vi "E_pressure_read_multiple_channels.vi"(3 "error in":errorcluster, 4 "Test Array":dbl[](array[numeric]), 5 "Test Mode":bool) -> (0 "error out":errorcluster, 1 "Scaled Pressures":dbl[](array[numeric]))   [LabVIEW 2013]
uses:
  <vilib>/DAQmx/read.llb/DAQmx Read (Analog 1D Wfm NChan NSamp).vi
  <vilib>/Analysis/baseanly.llb/Mean (DBL).vi
  <vilib>/DAQmx/miscellaneous.llb/DAQmx Fill In Error Info.vi
  <vilib>/Analysis/NI_AALBase.lvlib
panel:
  out "Raw Input Voltage":dbl[](array[numeric])
  out "data":waveform(dbl)[](graph)
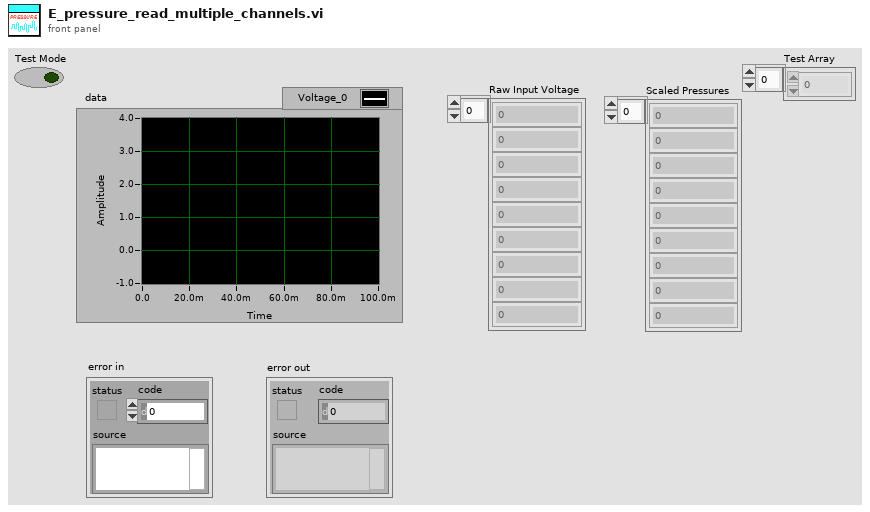
[diagram p1: front panel]
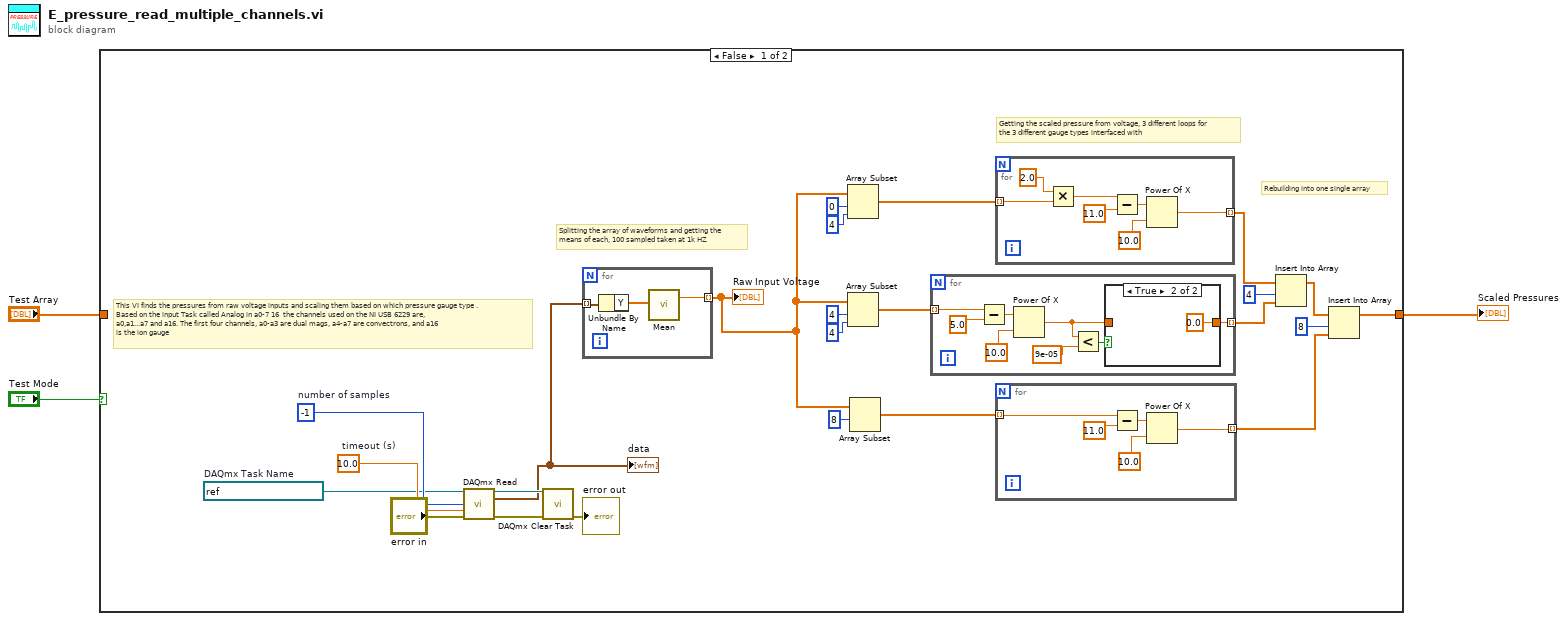
[diagram p0: block diagram]
diagram:
  n1 = case shown="False" "Test Mode" {
    tunnel: [w7 w53] -> w3
    tunnel: "Test Array" -> [_ w53]
    frame False {
      w23 = refnum<k21> "Analog in a0-7 16"  # DAQmx Task Name
      w26 = 10.0  # timeout (s)
      w27 = -1  # number of samples
      # "Rebuilding into one single array"
      # "Splitting the array of waveforms and getting the\nmeans of each, 100 sampled taken at 1k HZ"
      # "Getting the scaled pressure from voltage, 3 different loops for\nthe 3 different gauge types interfaced with"
      # "This VI finds the pressures from raw voltage inputs and scaling them based on which pressure gauge type .\nBased on the input Task called Analog in a0-7 16  the channels used on the NI USB 6229 are,\na0,a1...a7 and a16. The first four channels, a0-a3 are dual mags, a4-a7 are convectrons, and a16\nis the ion gauge"
      n2 = call-poly <vilib>:"DAQmx Read.vi"("task/channels in"=w23, "number of samples per channel"=w27, "timeout"=w26, "error in"="error in") -> ("task out"=w24:refnum<k21>, "data"=w22:waveform(dbl)[], "error out"=w25:errorcluster)  [unwired: 9 in]
      "data" <- w22
      n3 = call <vilib>:"DAQmx Clear Task.vi"("task in"=w24, "error in"=w25) -> ("error out"=→"error out":errorcluster)  [unwired: 13 in]
      n4 = for {
        tunnel: w22 -> [w51] mode=indexing
        tunnel: [w50] -> w6 mode=indexing
        n5 = Unbundle By Name(w51) -> ("Y"=w52:dbl[])
        n6 = call-poly <vilib>:"Mean.vi"("X"=w52) -> ("mean"=w50:dbl)  [unwired: 1 out]
      }
      "Raw Input Voltage" <- w6
      n7 = Array Subset(array=w6, index=0, length=4) -> (w19:dbl[])
      n8 = Array Subset(array=w6, index=4, length=4) -> (w15:dbl[])
      n9 = Array Subset(array=w6, index=8) -> (w14:dbl[])  [unwired: 1 in]
      n10 = for {
        tunnel: w15 -> [w37] mode=indexing
        tunnel: [w34] -> w11 mode=indexing
        n11 = Subtract(x=w37, y=5.0) -> (x-y=w39:dbl)
        n12 = Power Of X(1:10.0 ("y"), 2:w39) -> (0:w33:dbl)
        n13 = Less?(x=w33, y=9e-05) -> (x < y?=w35:bool)
        n14 = case shown="True" w35 {
          tunnel: [w41 0.0] -> w34
          tunnel: w33 -> [w41 _]
          frame False {
          }
          frame True {
          }
        }
      }
      n15 = for {
        tunnel: w19 -> [w45] mode=indexing
        tunnel: [w44] -> w13 mode=indexing
        n16 = Multiply(x=2.0, y=w45) -> (x*y=w49:dbl)
        n17 = Subtract(x=w49, y=11.0) -> (x-y=w47:dbl)
        n18 = Power Of X(1:10.0 ("y"), 2:w47) -> (0:w44:dbl)
      }
      n19 = for {
        tunnel: w14 -> [w29] mode=indexing
        tunnel: [w28] -> w9 mode=indexing
        n20 = Subtract(x=w29, y=11.0) -> (x-y=w31:dbl)
        n21 = Power Of X(1:10.0 ("y"), 2:w31) -> (0:w28:dbl)
      }
      n22 = Insert Into Array(array=w13, index=4, new element=w11) -> (w10:dbl[])
      n23 = Insert Into Array(array=w10, index=8, new element=w9) -> (w7:dbl[])
    }
    frame True {
    }
  }
  "Scaled Pressures" <- w3
